vi "GetStatus.vi"(6 "Stat Bin":refnum<vi>, 8 "error in (no error)":errorcluster, 11 "QuickSilver in":refnum<class "QuickSilver.lvclass">) -> (0 "error out":errorcluster, 2 "Status":i32, 3 "QuickSilver out":refnum<class "QuickSilver.lvclass">)   [LabVIEW 2012, in "QuickSilver.lvclass"]
uses:
  QuickSilver.lvclass
  QuickSilver.lvclass/QuickSilver.ctl
panel:
  # "Int"
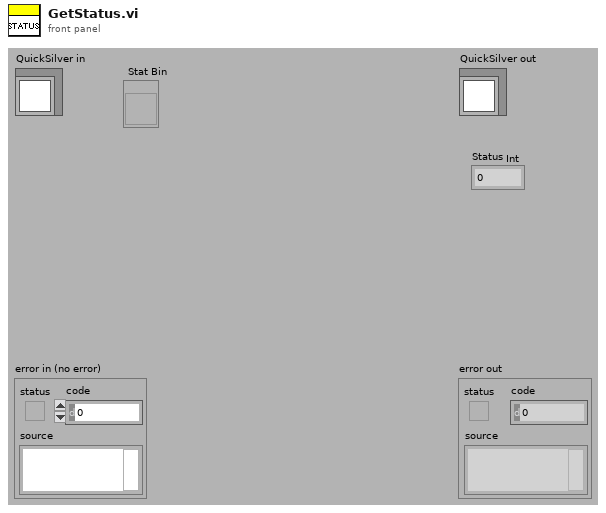
[diagram p1: front panel]
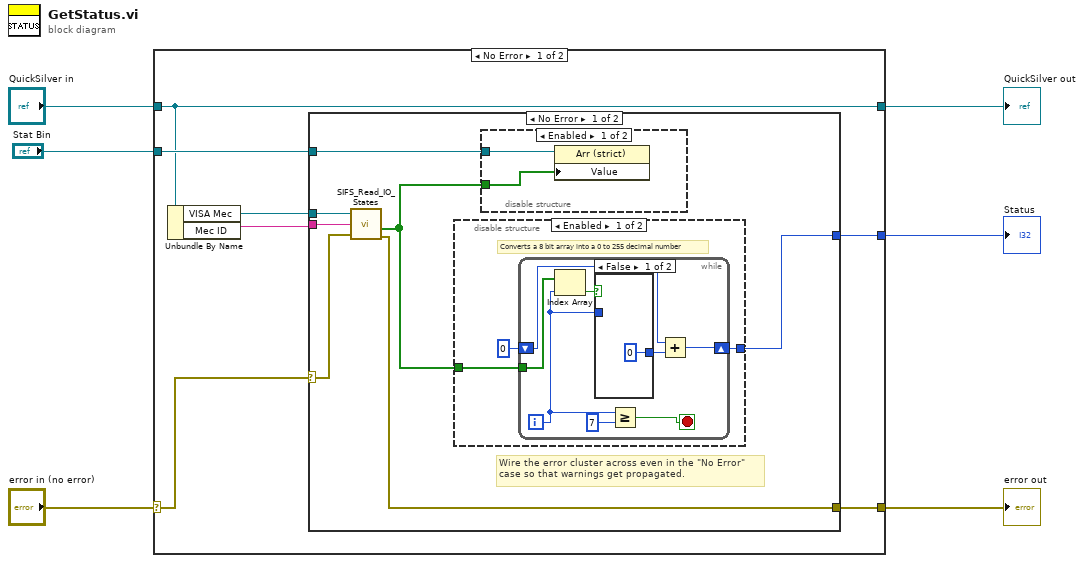
[diagram p0: block diagram]
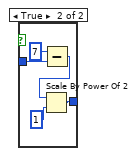
[diagram p3: hidden frame]
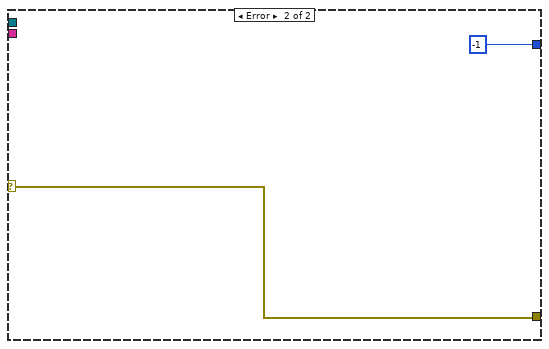
[diagram p5: hidden frame]
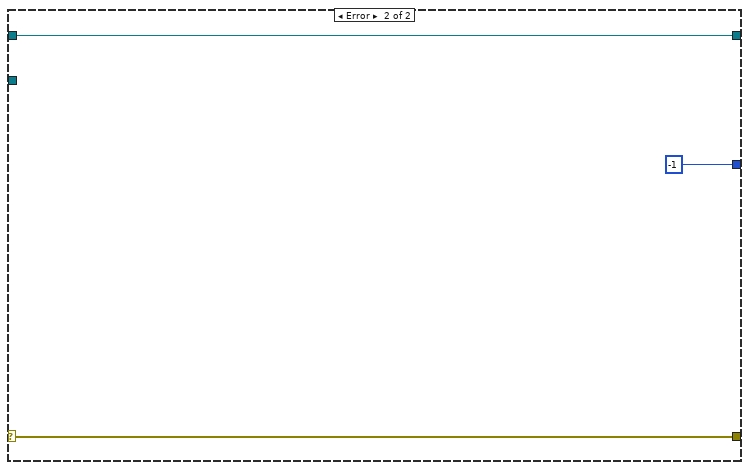
[diagram p6: hidden frame]
diagram:
  n1 = case shown="No Error" "error in (no error)" {
    selector: "error in (no error)" -> [w10 w44]
    tunnel: [w13 w44] -> w3
    tunnel: [w9 w43] -> w6
    tunnel: "QuickSilver in" -> [w9 w43]
    tunnel: [w12 -1] -> w2
    tunnel: "Stat Bin" -> [w11 _]
    frame No Error {
      n2 = Unbundle By Name(w9) -> ("VISA Mec"=w8:refnum<visa-resource-name>, "Mec ID"=w7:string)
      n3 = case shown="No Error" w10 {
        selector: w10 -> [w17 w41]
        tunnel: [w16 w41] -> w13
        tunnel: [w20 -1] -> w12
        tunnel: w7 -> [w19 _]
        tunnel: w8 -> [w18 _]
        tunnel: w11 -> [w14 _]
        frame No Error {
          # "Wire the error cluster across even in the \"No Error\"\ncase so that warnings get propagated."
          n4 = call "SIFS_Read_IO_States.vi"("VISA Name In"=w18, "ID"=w19, "error in"=w17) -> ("Status Byte"=w15:bool[], "error out"=w16:errorcluster)  [unwired: 4 out]
          n5 = disable-structure shown="Enabled" {
            disable-tunnel: [w24 _] -> w20
            disable-tunnel: w15 -> [w23 _]
            frame Enabled {
              # "Converts a 8 bit array into a 0 to 255 decimal number"
              n6 = while {
                tunnel: w23 -> [w33]
                shift-right: [w31] -> w24
                shift-left: 0 -> [w29]
                i -> [w26]
                stop <- w27 stop-if-true
                n7 = Index Array(array=w33, index=w26) -> (element=w32:bool)
                n8 = case shown="False" w32 {
                  tunnel: w26 -> [_ w39]
                  tunnel: [0 w35] -> w30
                  frame False {
                  }
                  frame True {
                    n9 = Subtract(x=7, y=w39) -> (x-y=w37:i32)
                    n10 = Scale By Power Of 2(n=w37, x=1) -> (x*2^n=w35:i32)
                  }
                }
                n11 = Greater Or Equal?(x=w26, y=7) -> (x >= y?=w27:bool)
                n12 = Add(x=w29, y=w30) -> (x+y=w31:i32)
              }
            }
            frame Disabled {
            }
          }
          n13 = disable-structure shown="Enabled" {
            disable-tunnel: w15 -> [w21 _]
            disable-tunnel: w14 -> [w22 _]
            frame Enabled {
              n14 = property class="Arr (strict)"(reference=w22, "Value"=w21) -> ()  [unwired: 1 in, 2 out]
            }
            frame Disabled {
            }
          }
        }
        frame Error {
        }
      }
    }
    frame Error {
    }
  }
  "error out" <- w3
  "QuickSilver out" <- w6
  "Status" <- w2
